vi "updateSettingValues.vi"(8 "error in (no error)":errorcluster, 11 "BaseSetting in":refnum<class "Setting.lvclass">) -> (0 "error out":errorcluster, 3 "BaseSetting out":refnum<class "Setting.lvclass">)   [LabVIEW 2016, in "Setting.lvclass"]
uses:
  Setting.lvclass
  Setting.lvclass/Setting.ctl
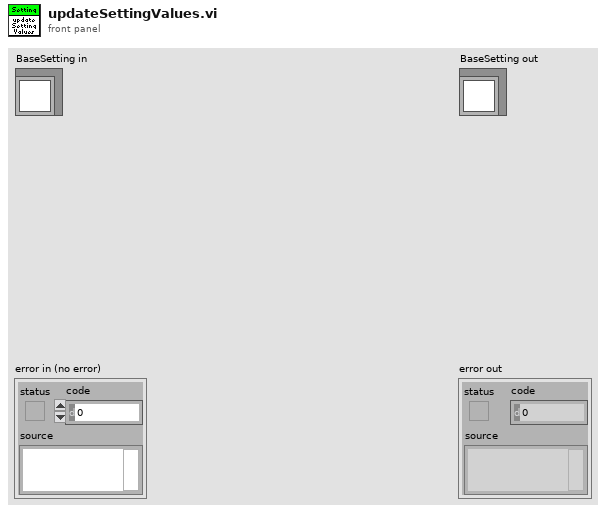
[diagram p1: front panel]
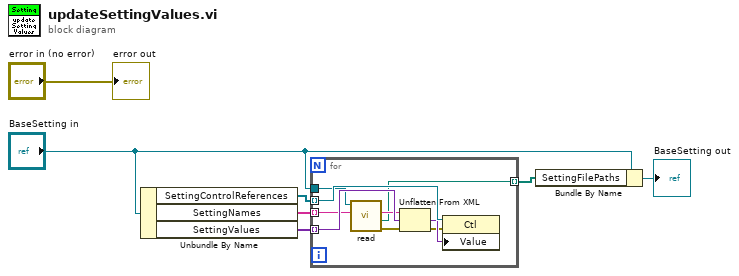
[diagram p0: block diagram]
diagram:
  n1 = Unbundle By Name("BaseSetting in") -> ("SettingControlReferences"=w7:refnum<vi>[], "SettingNames"=w6:string[], "SettingValues"=w5:variant[])
  n2 = for {
    tunnel: w6 -> [w12] mode=indexing
    tunnel: w5 -> [w16] mode=indexing
    tunnel: w7 -> [w15] mode=indexing
    tunnel: [w8] -> w3 mode=indexing
    tunnel: "BaseSetting in" -> [w9]
    n3 = call "read.vi"("Name"=w12, "BaseSetting in"=w9) -> ("error out"=w11:errorcluster, "SettingFilePath"=w8:path, "XML"=w10:string)  [unwired: 6 in, 1 out]
    n4 = Unflatten From XML(xml string=w10, type=w16, error in (no error)=w11) -> (value=w14:variant, error out=w13:errorcluster)
    n5 = property class="Ctl"(reference=w15, error in=w13, "Value"=w14) -> ()  [unwired: 2 out]
  }
  n6 = Bundle By Name(cluster="BaseSetting in", "SettingFilePaths"=w3) -> (→"BaseSetting out":refnum<class "Setting.lvclass">)
  "error out" <- "error in (no error)"
